vi "Detect unsuported Brick and fall and keep track.vi"(7 "Dropped Set":set{i32}(c389), 10 "Grid":i32[][][](array[numeric]), 11 "Brick Map":map{i32, T1[]}(c390)) -> (1 "Continue":bool, 2 "Grid out":i32[][][](array[numeric]), 3 "Brick Map":map{i32, T1[]}(c390), 5 "Dropped Set":set{i32}(c389))   [LabVIEW 2023]
uses:
  Cluster_Node.ctl
panel:
  out "left":i32
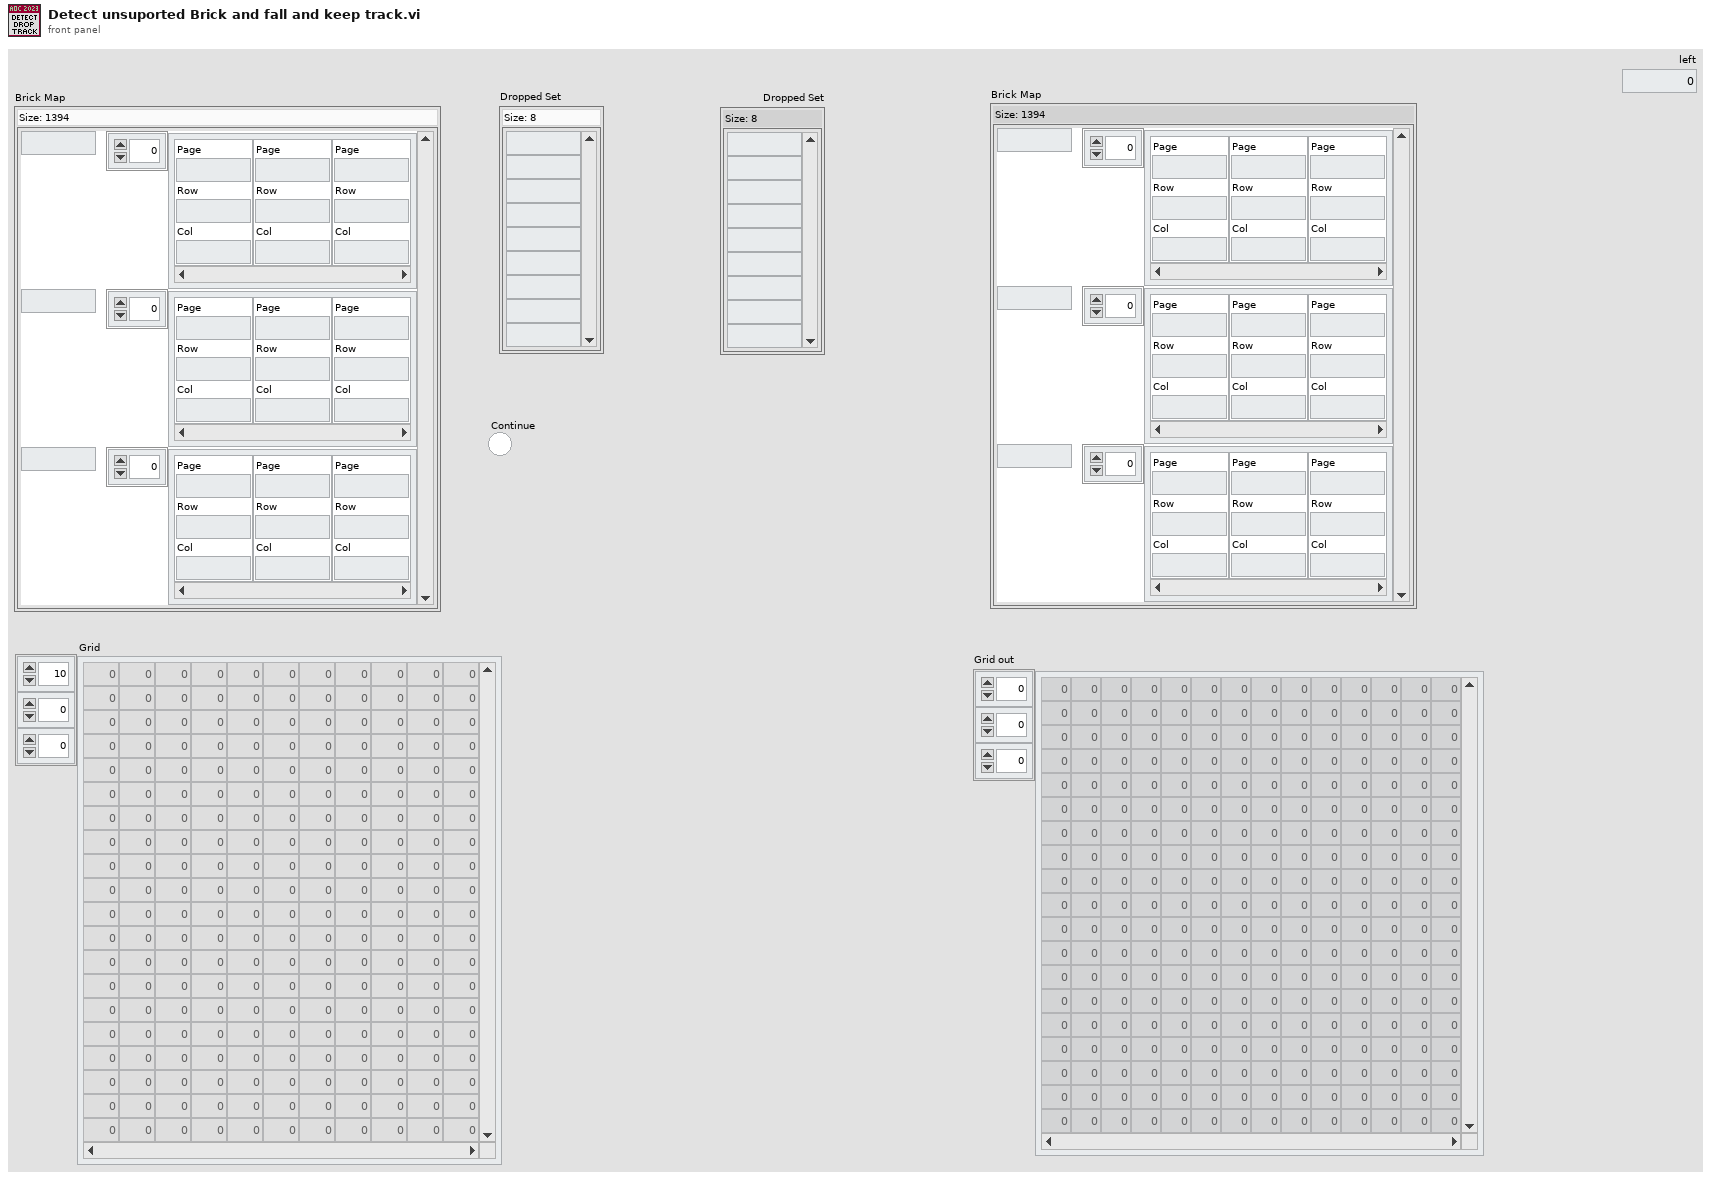
[diagram p1: front panel]
types:
  T1 = typedef "Cluster_Node.ctl" = cluster{"Page":i32, "Row":i32, "Col":i32}
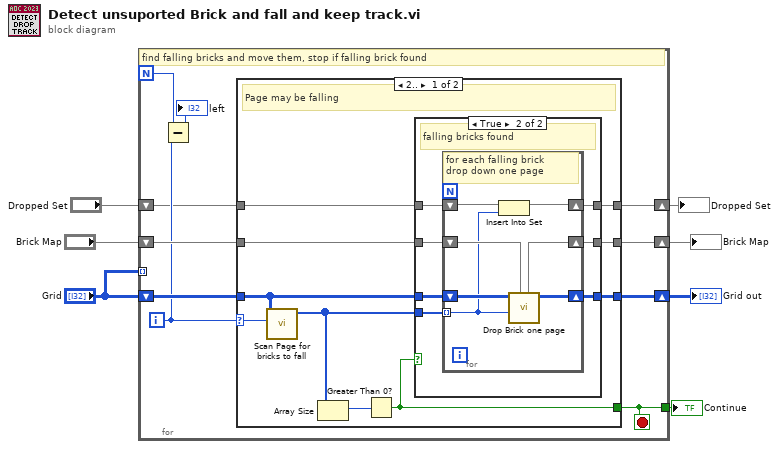
[diagram p0: block diagram]
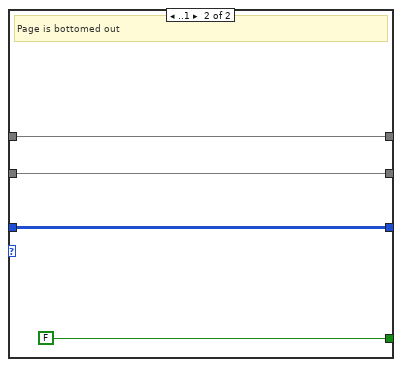
[diagram p3: hidden frame]
diagram:
  n1 = for {
    N -> [w12]
    shift-right: [w14] -> w5
    shift-left: "Grid" -> [w15]
    shift-right: [w16] -> w4
    shift-left: "Brick Map" -> [w17]
    tunnel: [w13] -> w6
    tunnel: "Grid" -> [_] mode=indexing
    shift-right: [w8] -> w1
    shift-left: "Dropped Set" -> [w9]
    i -> [w11]
    stop <- w13 stop-if-true
    # "find falling bricks and move them, stop if falling brick found"
    n2 = Subtract(x=w12, y=w11) -> (x-y=→"left":i32)
    n3 = case shown="2.." w11 {
      selector: w11 -> [w27 _]
      tunnel: [w25 FALSE] -> w13
      tunnel: w17 -> [w24 w48]
      tunnel: [w22 w48] -> w16
      tunnel: w15 -> [w23 w47]
      tunnel: [w21 w47] -> w14
      tunnel: w9 -> [w19 w45]
      tunnel: [w18 w45] -> w8
      frame 2.. {
        # "Page may be falling"
        n4 = call "Scan Page for bricks to fall.vi"("Page Index"=w27, "Block Array"=w23) -> ("Fall IDs"=w20:i32[])  [unwired: 9 in]
        n5 = Array Size(array=w20) -> (size(s)=w26:i32)
        n6 = Greater Than 0?(x=w26) -> (x > 0?=w25:bool)
        n7 = case shown="True" w25 {
          tunnel: w24 -> [w30 w36]
          tunnel: w23 -> [w29 w34]
          tunnel: [w30 w35] -> w22
          tunnel: [w29 w33] -> w21
          tunnel: w20 -> [_ w37]
          tunnel: w19 -> [w28 w32]
          tunnel: [w28 w31] -> w18
          frame False {
            # "no falling bricks detected"
          }
          frame True {
            # "falling bricks found"
            n8 = for {
              tunnel: w37 -> [w38] mode=indexing
              shift-right: [w43] -> w35
              shift-left: w36 -> [w44]
              shift-right: [w41] -> w33
              shift-left: w34 -> [w42]
              shift-right: [w39] -> w31
              shift-left: w32 -> [w40]
              # "for each falling brick\ndrop down one page"
              n9 = Insert Into Set(10:w38, 11:w40) -> (3:w39:set{i32})  [unwired: 1 out]
              n10 = call "Drop Brick one page.vi"("Map in"=w44, "ID"=w38, "Array in"=w42) -> ("Array out"=w41:i32[][][], "Map out"=w43:map{i32, T1[]})  [unwired: 7 in]
            }
          }
        }
      }
      frame ..1 {
        # "Page is bottomed out"
      }
    }
  }
  "Continue" <- w6
  "Grid out" <- w5
  "Brick Map" <- w4
  "Dropped Set" <- w1
